vi "Frame Rate.vi"(11 "Test Case In":refnum<class "Test.Camera.lvclass">) -> (0 "error out":errorcluster, 3 "Test Case Out":refnum<class "Test.Camera.lvclass">)   [LabVIEW 2020, in "Test.Camera.lvclass"]
uses:
  Test.Camera.lvclass
  C:/Program Files (x86)/National Instruments/LabVIEW 2020/vi.lib/Astemes/LUnit/Test Case.lvclass
  g_industrial_cam/Camera/Camera.lvclass/Camera.ctl
  <vilib>/Astemes/LUnit/Test Case.lvclass/Test Case.ctl
  c3e2611f-c54f-4219-a549-b8da21c7f085.vi
  0aa1576c-e916-4ad0-9a97-64bd3e4eb69b.vi
  759e5037-5df0-4144-95b6-409846063909.vi
  g_industrial_cam/Camera/GetSetFrameRate.vi
  g_industrial_cam/Camera/GetSetFrameRateEnable.vi
  <vilib>/Astemes/LUnit/Append Pass Result.vi
  <vilib>/Astemes/LUnit/Append Fail Result.vi
  <vilib>/Astemes/LUnit/Describe Comparison.vi
  0aa1576c-e916-4ad0-9a97-64bd3e4eb69b.vi/9c5d11cd-9439-4240-a1ee-d9baace9c924.vi
  759e5037-5df0-4144-95b6-409846063909.vi/9c5d11cd-9439-4240-a1ee-d9baace9c924.vi
  <vilib>/Astemes/LUnit/Run In UI.vi
  <vilib>/Utility/error.llb/Clear Errors.vi
  g_industrial_cam/Camera/Check Not Disconnected.vi
  <vilib>/Utility/error.llb/Error Cluster From Error Code.vi
  <vilib>/Astemes/LUnit/Describe Variant.vi
  <vilib>/Astemes/LUnit/Test Case.lvclass
  g_industrial_cam/Camera/Camera.lvclass
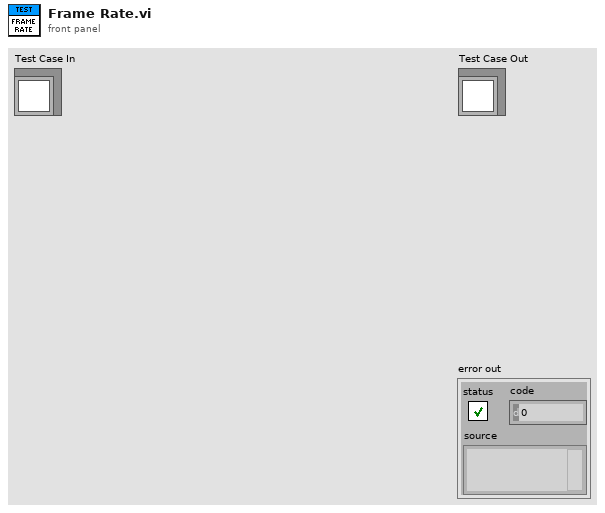
[diagram p1: front panel]
types:
  T1 = enum16{"Get Values", "Set Frame Rate", "Enable Frame Rate"}
  T2 = enum16{"Get Values", "Set Frame Rate", "Enable Frame Rate"}[]
  T3 = cluster{"Enabled":bool, "Min":dbl, "Max":dbl, "Frame Rate":dbl, "Avaliable":bool}
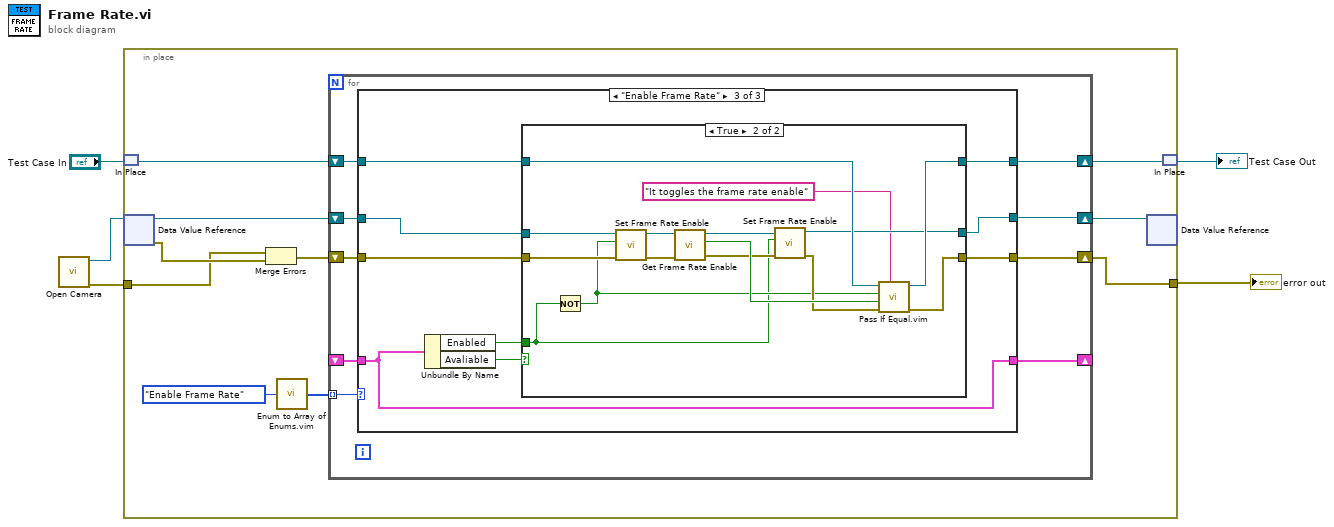
[diagram p0: block diagram]
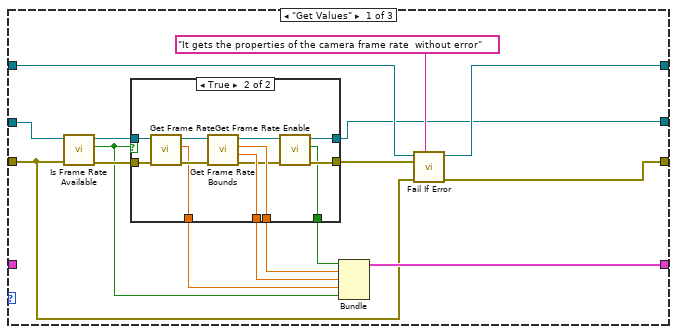
[diagram p2: hidden frame]
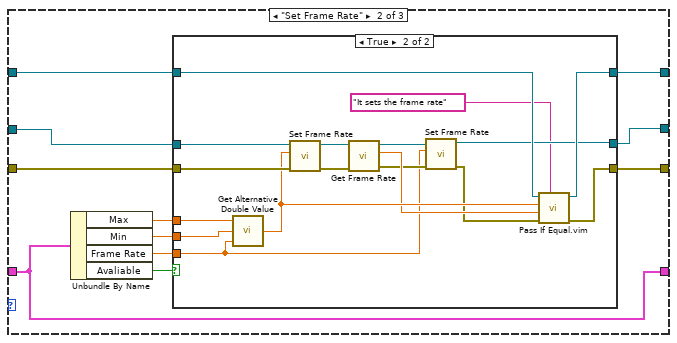
[diagram p4: hidden frame]
diagram:
  n1 = call "Open Camera.vi"() -> ("error out"=w5:errorcluster, "Camera"=w4:refnum<data-value>)  [unwired: 10 in]
  n2 = in-place {
    in-place-border: w5 -> [w8]
    in-place-border: [w7] -> w2
    n3 = in-place-match #1("Test Case In") -> (w10:refnum<class "Test.Camera.lvclass">)
    n4 = in-place-dvr #2(w4) -> (w14:refnum<class "Camera.lvclass">, w15:errorcluster)
    n5 = Merge Errors(w8, w15) -> (w13:errorcluster)
    n6 = call "Enum to Array of Enums.vim"("enum"=T1."Enable Frame Rate") -> ("array of enums"=w11:T2)
    n7 = for {
      tunnel: w11 -> [w22] mode=indexing
      shift-right: [w21] -> w9
      shift-left: w14 -> [w24]
      shift-right: [w20] -> _
      shift-left: _ -> [w19]
      shift-right: [w17] -> w6
      shift-left: w10 -> [w18]
      shift-right: [w16] -> w7
      shift-left: w13 -> [w23]
      n8 = case shown="\"Enable Frame Rate\"" w22 {
        tunnel: w24 -> [w35 w64 w93]
        tunnel: w23 -> [w34 w65 w94]
        tunnel: [w26 w57 w88] -> w21
        tunnel: [w36 w55 w86] -> w20
        tunnel: w19 -> [_ w55 w86]
        tunnel: w18 -> [w40 w59 w90]
        tunnel: [w39 w58 w89] -> w17
        tunnel: [w37 w56 w87] -> w16
        frame "Get Values" {
          n9 = call "Is Frame Rate Available.vi"("error in (no error)"=w34, "Camera in"=w35) -> ("error out"=w33:errorcluster, "Avaliable"=w32:bool, "Camera"=w31:refnum<class "Camera.lvclass">)  [unwired: 7 in]
          n10 = case shown="True" w32 {
            tunnel: w33 -> [w41 w53]
            tunnel: w31 -> [w42 w54]
            tunnel: [_ w49] -> w30
            tunnel: [_ w48] -> w29
            tunnel: [_ w46] -> w28
            tunnel: [w41 w44] -> w27
            tunnel: [w42 w47] -> w26
            tunnel: [_ w43] -> w25
            frame False {
            }
            frame True {
              n11 = call "Get Frame Rate.vi"("error in (no error)"=w53, "Camera in"=w54) -> ("error out"=w52:errorcluster, "Frame Rate"=w49:dbl, "Camera"=w51:refnum<class "Camera.lvclass">)  [unwired: 7 in]
              n12 = call "Get Frame Rate Bounds.vi"("error in (no error)"=w52, "Camera in"=w51) -> ("error out"=w45:errorcluster, "Max"=w48:dbl, "Min"=w46:dbl, "Camera"=w50:refnum<class "Camera.lvclass">)  [unwired: 6 in]
              n13 = call "Get Frame Rate Enable.vi"("error in (no error)"=w45, "Camera in"=w50) -> ("error out"=w44:errorcluster, "Enabled"=w43:bool, "Camera"=w47:refnum<class "Camera.lvclass">)  [unwired: 7 in]
            }
          }
          n14 = Bundle("Enabled"=w25, "Min"=w28, "Max"=w29, "Frame Rate"=w30, "Avaliable"=w32) -> (w36:T3)  [unwired: 1 in]
          n15 = call <vilib>:"Fail If Error.vi"("Description"="It gets the properties of the camera frame rate  without error", "error in (no error)"=w34, "Assert error"=w27, "LUnit Test Case In"=w40) -> ("error out"=w37:errorcluster, "LUnit Test Case Out"=w39:refnum<class "Test.Camera.lvclass">)  [unwired: 6 in]
        }
        frame "Set Frame Rate" {
          n16 = Unbundle By Name(w55) -> ("Max"=w62:dbl, "Min"=w61:dbl, "Frame Rate"=w60:dbl, "Avaliable"=w63:bool)
          n17 = case shown="True" w63 {
            tunnel: w65 -> [w68 w80]
            tunnel: w64 -> [w67 w79]
            tunnel: w62 -> [_ w85]
            tunnel: w61 -> [_ w84]
            tunnel: w60 -> [_ w72]
            tunnel: w59 -> [w66 w81]
            tunnel: [w66 w82] -> w58
            tunnel: [w67 w70] -> w57
            tunnel: [w68 w83] -> w56
            frame False {
            }
            frame True {
              n18 = call "Get Alternative Double Value.vi"("Value"=w72, "Min"=w84, "Max"=w85) -> ("Alternative Value"=w78:dbl)  [unwired: 1 in]
              n19 = call "Set Frame Rate.vi"("error in (no error)"=w80, "Frame Rate"=w78, "Camera in"=w79) -> ("error out"=w77:errorcluster, "Camera"=w76:refnum<class "Camera.lvclass">)  [unwired: 7 in]
              n20 = call "Get Frame Rate.vi"("error in (no error)"=w77, "Camera in"=w76) -> ("error out"=w74:errorcluster, "Frame Rate"=w75:dbl, "Camera"=w73:refnum<class "Camera.lvclass">)  [unwired: 7 in]
              n21 = call "Set Frame Rate.vi"("error in (no error)"=w74, "Frame Rate"=w72, "Camera in"=w73) -> ("error out"=w71:errorcluster, "Camera"=w70:refnum<class "Camera.lvclass">)  [unwired: 7 in]
              n22 = call "Pass If Equal.vim"("Description"="It sets the frame rate", "error in (no error)"=w71, "Actual"=w75, "Expected"=w78, "LUnit Test Case In"=w81) -> ("error out"=w83:errorcluster, "LUnit Test Case Out"=w82:refnum<class "Test.Camera.lvclass">)  [unwired: 5 in]
            }
          }
        }
        frame "Enable Frame Rate" {
          n23 = Unbundle By Name(w86) -> ("Enabled"=w91:bool, "Avaliable"=w92:bool)
          n24 = case shown="True" w92 {
            tunnel: w94 -> [w97 w109]
            tunnel: w93 -> [w96 w108]
            tunnel: w91 -> [_ w98]
            tunnel: w90 -> [w95 w110]
            tunnel: [w95 w111] -> w89
            tunnel: [w96 w101] -> w88
            tunnel: [w97 w112] -> w87
            frame False {
            }
            frame True {
              n25 = Not(x=w98) -> (.not. x?=w99:bool)
              n26 = call "Set Frame Rate Enable.vi"("error in (no error)"=w109, "Enable"=w99, "Camera in"=w108) -> ("error out"=w107:errorcluster, "Camera"=w106:refnum<class "Camera.lvclass">)  [unwired: 7 in]
              n27 = call "Get Frame Rate Enable.vi"("error in (no error)"=w107, "Camera in"=w106) -> ("error out"=w104:errorcluster, "Enabled"=w105:bool, "Camera"=w103:refnum<class "Camera.lvclass">)  [unwired: 7 in]
              n28 = call "Set Frame Rate Enable.vi"("error in (no error)"=w104, "Enable"=w98, "Camera in"=w103) -> ("error out"=w102:errorcluster, "Camera"=w101:refnum<class "Camera.lvclass">)  [unwired: 7 in]
              n29 = call "Pass If Equal.vim"("Description"="It toggles the frame rate enable", "error in (no error)"=w102, "Actual"=w105, "Expected"=w99, "LUnit Test Case In"=w110) -> ("error out"=w112:errorcluster, "LUnit Test Case Out"=w111:refnum<class "Test.Camera.lvclass">)  [unwired: 5 in]
            }
          }
        }
      }
    }
    n30 = in-place-dvr #2(w9) -> ()  [unwired: 2 out]
    n31 = in-place-match #1(w6) -> (→"Test Case Out":refnum<class "Test.Camera.lvclass">)
  }
  "error out" <- w2
